vi "Z-axis travel safety interlock.vi"(7 "Interlock check type":T1, 8 "error in (no error)":errorcluster, 9 "Z Limit (+/- um)":sgl, 10 "Z move to":sgl, 11 "Z Current":sgl) -> (0 "error out":errorcluster, 3 "Z":sgl)   [LabVIEW 2020]
uses:
  Typedefs/Z intelock check type.ctl
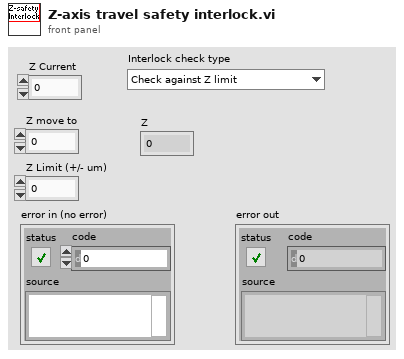
[diagram p1: front panel]
types:
  T1 = typedef "Z intelock check type.ctl" = enum16{"Check against Z limit", "Check againt current position"}
  T2 = cluster{"Caption-Right button":string, "Caption-Left button":string, "Message to display":string, "Delay before close":u32, "Window Colour":u32, "Cancel button disabled?":enum8{"Enabled", "Disabled", "Disabled and Grayed Out"}}
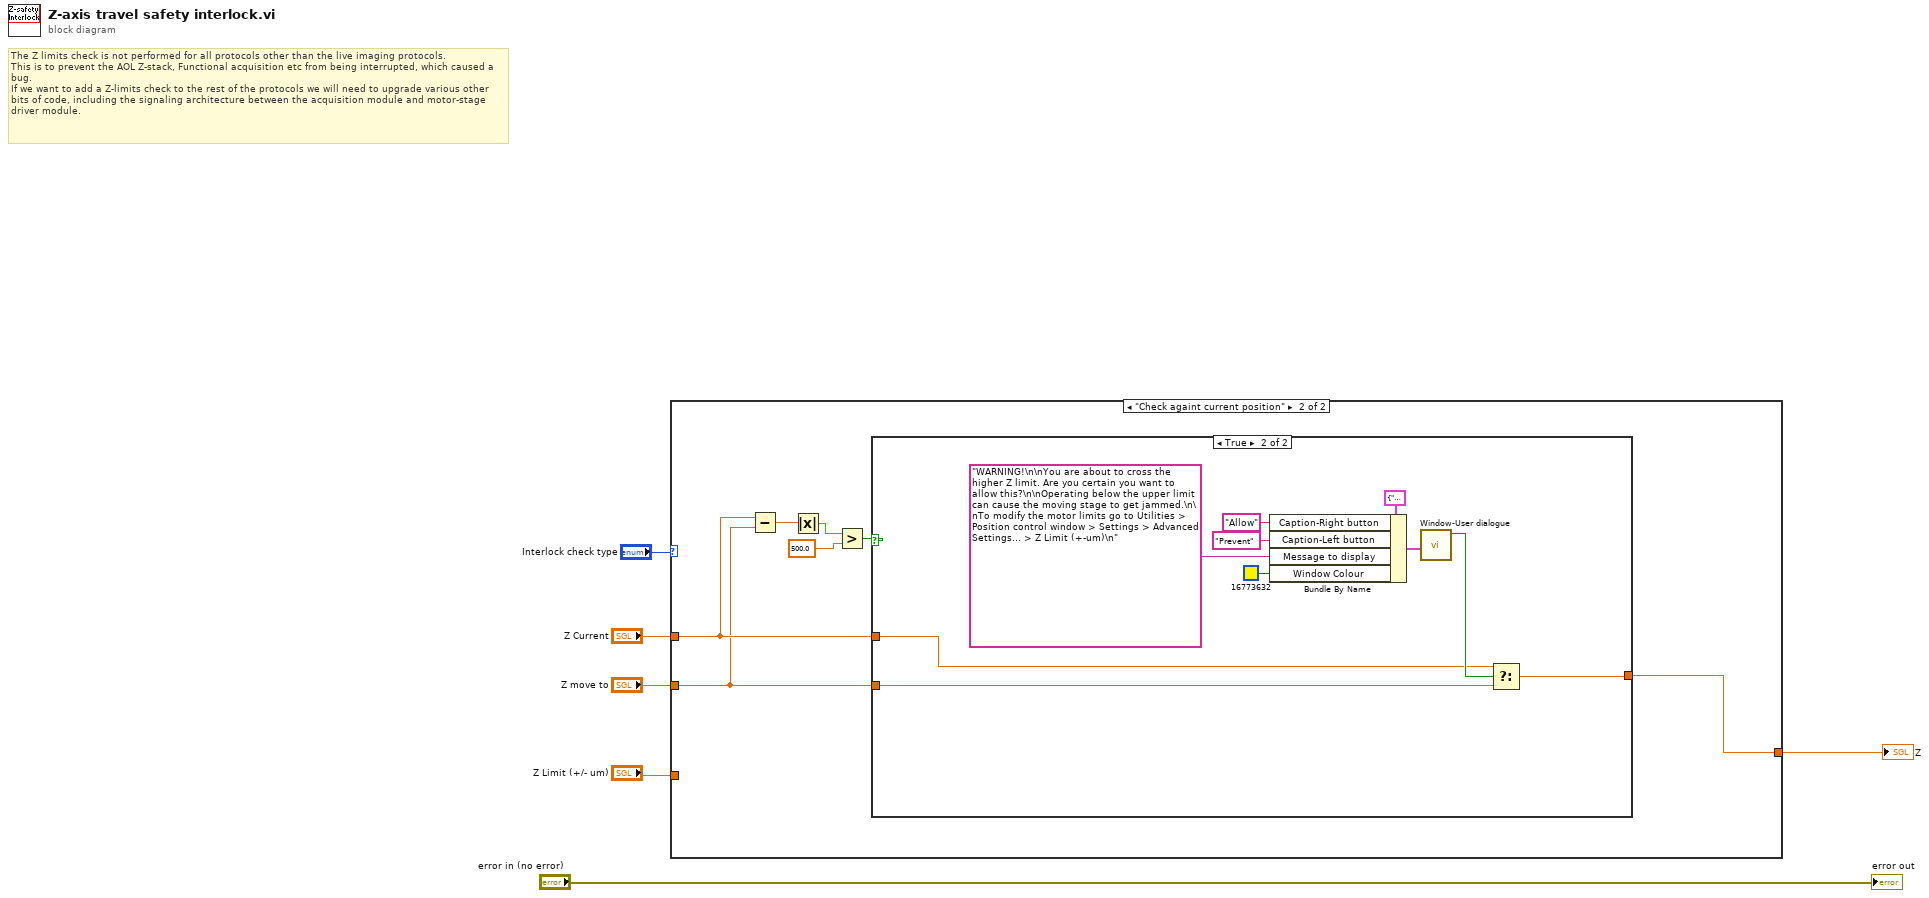
[diagram p0: block diagram]
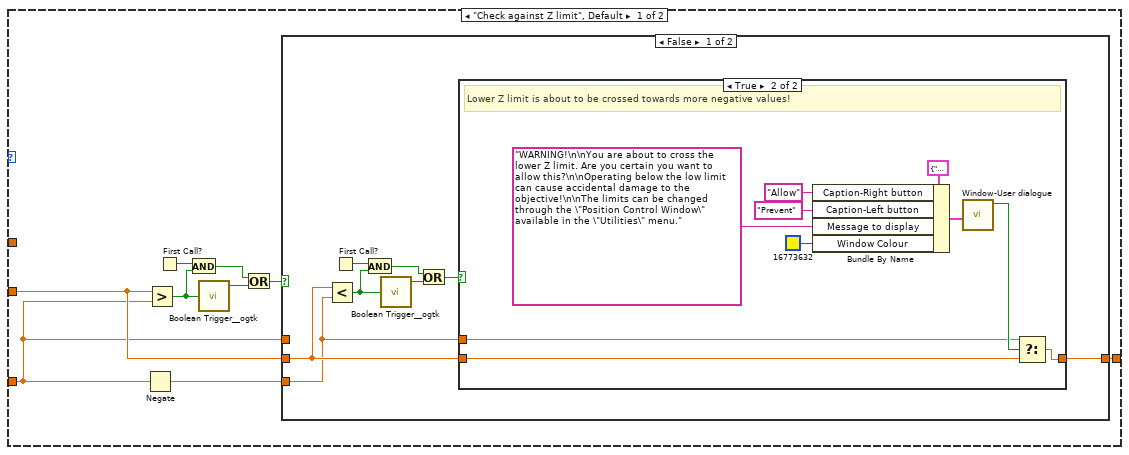
[diagram p2: hidden frame]
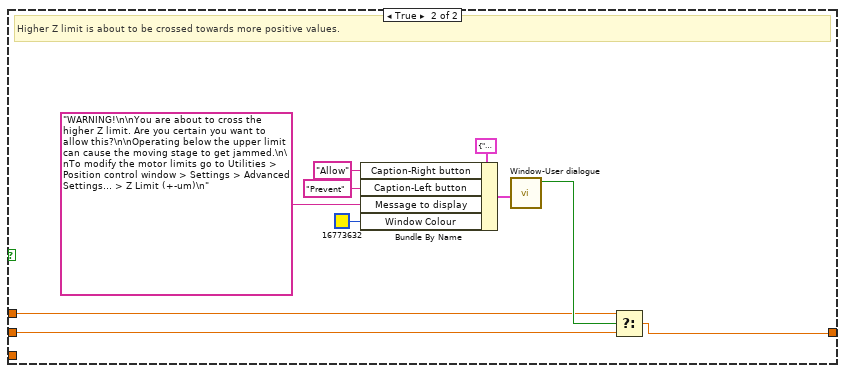
[diagram p4: hidden frame]
diagram:
  # "The Z limits check is not performed for all protocols other than the live imaging protocols.\nThis is to prevent the AOL Z-stack, Functional acquisition etc from being interrupted, which caused a bug.\nIf we want to add a Z-limits check to the rest of the protocols we will need to upgrade various other bits of code, including the signaling architecture between the acquisition module and motor-stage driver module."
  n1 = case shown="\"Check againt current position\"" "Interlock check type" {
    tunnel: [w15 w45] -> w6
    tunnel: "Z move to" -> [w14 w46]
    tunnel: "Z Current" -> [_ w47]
    tunnel: "Z Limit (+/- um)" -> [w7 _]
    frame "Check against Z limit", Default {
      n2 = Negate(x=w7) -> (-x=w13:sgl)
      n3 = Greater?(x=w14, y=w7) -> (0:w11:bool)
      n4 = First Call?() -> (First Call?: T/F=w12:bool)
      n5 = And(x=w12, y=w11) -> (x .and. y?=w9:bool)
      n6 = call <userlib>:"Boolean Trigger__ogtk.vi"("Boolean Input"=w11) -> ("Rising Edge"=w10:bool)  [unwired: 1 in, 1 out]
      n7 = Or(x=w9, y=w10) -> (x .or. y?=w8:bool)
      n8 = case shown="False" w8 {
        tunnel: w14 -> [w22 w44]
        tunnel: [w23 w43] -> w15
        tunnel: w7 -> [_ w41]
        tunnel: w13 -> [w21 _]
        frame False {
          n9 = Less?(x=w22, y=w21) -> (x < y?=w20:bool)
          n10 = First Call?() -> (First Call?: T/F=w19:bool)
          n11 = And(x=w19, y=w20) -> (x .and. y?=w16:bool)
          n12 = call <userlib>:"Boolean Trigger__ogtk.vi"("Boolean Input"=w20) -> ("Rising Edge"=w18:bool)  [unwired: 1 in, 1 out]
          n13 = Or(x=w16, y=w18) -> (x .or. y?=w17:bool)
          n14 = case shown="True" w17 {
            tunnel: w22 -> [w24 w34]
            tunnel: [w24 w33] -> w23
            tunnel: w21 -> [_ w31]
            frame False {
            }
            frame True {
              # "Lower Z limit is about to be crossed towards more negative values!"
              n15 = Bundle By Name(cluster=T2 {"Caption-Right button"="", "Caption-Left button"="", "Message to display"="", "Delay before close"=0, "Window Colour"=16448250, "Cancel button disabled?"=enum."Enabled"} ("Input cluster"), "Caption-Right button"="Allow", "Caption-Left button"="Prevent", "Message to display"="WARNING!\n\nYou are about to cross the lower Z limit. Are you certain you want to allow this?\n\nOperating below the low limit can cause accidental damage to the objective!\n\nThe limits can be changed through the \"Position Control Window\" available in the \"Utilities\" menu." ("Message string"), "Window Colour"=u32 16773632) -> (w26:T2)
              n16 = call "Window-User dialogue.vi"("Input cluster"=w26) -> ("Left Button (Cancel)"=w32:bool)  [unwired: 10 in]
              n17 = Select(t=w31, s=w32, f=w34) -> (s? t:f=w33:sgl)
            }
          }
        }
        frame True {
          # "Higher Z limit is about to be crossed towards more positive values."
          n18 = Bundle By Name(cluster=T2 {"Caption-Right button"="", "Caption-Left button"="", "Message to display"="", "Delay before close"=0, "Window Colour"=16448250, "Cancel button disabled?"=enum."Enabled"} ("Input cluster"), "Caption-Right button"="Allow", "Caption-Left button"="Prevent", "Message to display"="WARNING!\n\nYou are about to cross the higher Z limit. Are you certain you want to allow this?\n\nOperating below the upper limit can cause the moving stage to get jammed.\n\nTo modify the motor limits go to Utilities > Position control window > Settings > Advanced Settings… > Z Limit (+-um)\n" ("Message string"), "Window Colour"=u32 16773632) -> (w36:T2)
          n19 = call "Window-User dialogue.vi"("Input cluster"=w36) -> ("Left Button (Cancel)"=w42:bool)  [unwired: 10 in]
          n20 = Select(t=w41, s=w42, f=w44) -> (s? t:f=w43:sgl)
        }
      }
    }
    frame "Check againt current position" {
      n21 = Subtract(x=w47, y=w46) -> (x-y=w51:sgl)
      n22 = Absolute Value(x=w51) -> (abs(x)=w50:sgl)
      n23 = Greater?(x=w50, y=sgl 500.0) -> (0:w48:bool)
      n24 = case shown="True" w48 {
        tunnel: w47 -> [_ w55]
        tunnel: w46 -> [w52 w54]
        tunnel: [w52 w53] -> w45
        frame False {
        }
        frame True {
          n25 = Bundle By Name(cluster=T2 {"Caption-Right button"="", "Caption-Left button"="", "Message to display"="", "Delay before close"=0, "Window Colour"=16448250, "Cancel button disabled?"=enum."Enabled"} ("Input cluster"), "Caption-Right button"="Allow", "Caption-Left button"="Prevent", "Message to display"="WARNING!\n\nYou are about to cross the higher Z limit. Are you certain you want to allow this?\n\nOperating below the upper limit can cause the moving stage to get jammed.\n\nTo modify the motor limits go to Utilities > Position control window > Settings > Advanced Settings… > Z Limit (+-um)\n" ("Message string"), "Window Colour"=u32 16773632) -> (w58:T2)
          n26 = call "Window-User dialogue.vi"("Input cluster"=w58) -> ("Left Button (Cancel)"=w56:bool)  [unwired: 10 in]
          n27 = Select(t=w55, s=w56, f=w54) -> (s? t:f=w53:sgl)
        }
      }
    }
  }
  "Z" <- w6
  "error out" <- "error in (no error)"
